vi "Configure Segment Independence.vi"(0 "VISA resource name":refnum<visa-resource-name>, 1 "Enable Independent Sweep Time (F: Disable)":bool, 2 "Enable Arbitrary Segment (F: Disable)":bool, 5 "Channel (1)":i32=1, 7 "Enable Independent IF Bandwidth (F: Disable)":bool, 9 "Enable Independent Power Level (F: Disable)":bool, 11 "error in (no error)":errorcluster, 12 "Enable X-axis Spacing (F: Disable)":bool) -> (4 "VISA resource name out":refnum<visa-resource-name>, 15 "error out":errorcluster)   [LabVIEW 2018, in "Keysight PNA Series.lvlib"]
doc: "Configures whether some properties can be set independently for each segment."
uses:
  Keysight PNA Series.lvlib
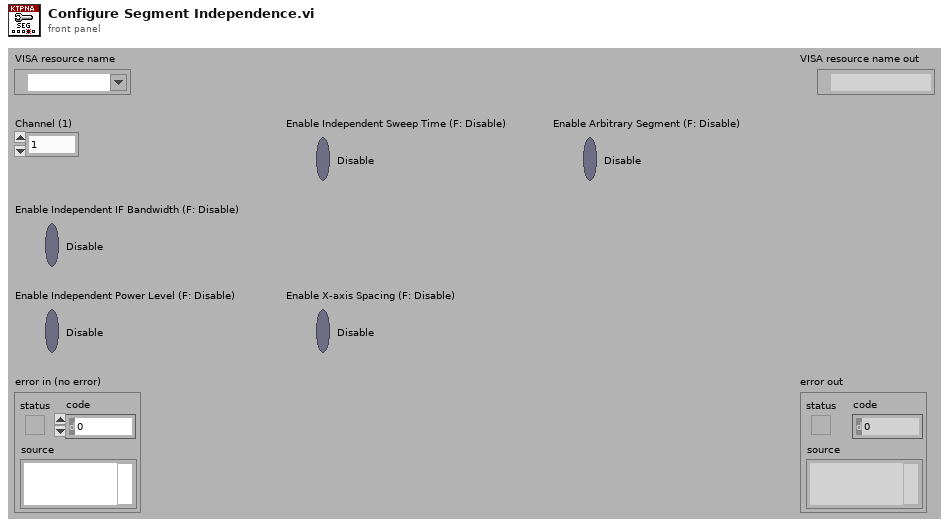
[diagram p1: front panel]
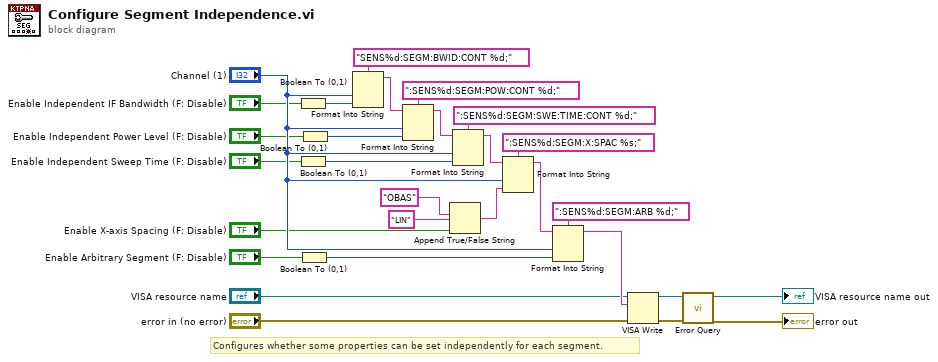
[diagram p0: block diagram]
diagram:
  # "Configures whether some properties can be set independently for each segment."
  n1 = Boolean To (0,1)(Boolean="Enable Independent IF Bandwidth (F: Disable)") -> (0, 1=w12:i16)
  n2 = Boolean To (0,1)(Boolean="Enable Independent Sweep Time (F: Disable)") -> (0, 1=w7:i16)
  n3 = Boolean To (0,1)(Boolean="Enable Arbitrary Segment (F: Disable)") -> (0, 1=w5:i16)
  n4 = Boolean To (0,1)(Boolean="Enable Independent Power Level (F: Disable)") -> (0, 1=w9:i16)
  n5 = Format Into String(format string="SENS%d:SEGM:BWID:CONT %d;", "Channel (1)", w12) -> (resulting string=w27:string)  [unwired: 2 in, 1 out]
  n6 = Format Into String(format string=":SENS%d:SEGM:POW:CONT %d;", initial string=w27, "Channel (1)", w9) -> (resulting string=w25:string)  [unwired: 1 in, 1 out]
  n7 = Append True/False String(1:"Enable X-axis Spacing (F: Disable)", 2:"LIN" ("true string"), 3:"OBAS" ("true string")) -> (0:w1:string)  [unwired: 1 in]
  n8 = Format Into String(format string=":SENS%d:SEGM:SWE:TIME:CONT %d;", initial string=w25, "Channel (1)", w7) -> (resulting string=w23:string)  [unwired: 1 in, 1 out]
  n9 = Format Into String(format string=":SENS%d:SEGM:X:SPAC %s;", initial string=w23, "Channel (1)", w1) -> (resulting string=w21:string)  [unwired: 1 in, 1 out]
  n10 = Format Into String(format string=":SENS%d:SEGM:ARB %d;", initial string=w21, "Channel (1)", w5) -> (resulting string=w19:string)  [unwired: 1 in, 1 out]
  n11 = VISA Write(VISA resource name="VISA resource name", write buffer=w19, error in (no error)="error in (no error)") -> (VISA resource name out=w16:refnum<visa-resource-name>, error out=w15:errorcluster)  [unwired: 1 out]
  n12 = call "Error Query.vi"("error in (no error)"=w15, "VISA resource name"=w16) -> ("error out"=→"error out":errorcluster, "VISA resource name out"=→"VISA resource name out":refnum<visa-resource-name>)  [unwired: 6 in, 2 out]
